vi "setTimebase.vi"(8 "error in (no error)":errorcluster, 9 "Delay [s]":dbl, 10 "Timebase [s/Div]":dbl, 11 "ScopeKeysight in":refnum<class "ScopeKeysight.lvclass">) -> (0 "error out":errorcluster, 3 "ScopeKeysight out":refnum<class "ScopeKeysight.lvclass">)   [LabVIEW 2023, in "ScopeKeysight.lvclass"]
doc: "<b>Author:</b> Wolfgang\n<b>Description:</b> Configure the timebase"
uses:
  ScopeKeysight.lvclass
  ScopeKeysight.lvclass/ScopeKeysight.ctl
  Driver/Public/Configure/Configure Timebase (Basic).vi
  Driver/Keysight-DSQx3014T.lvlib
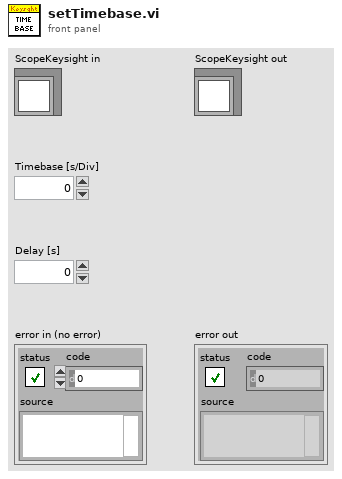
[diagram p1: front panel]
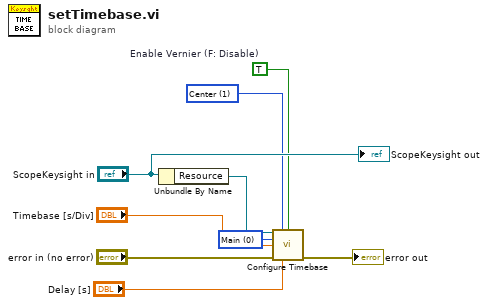
[diagram p0: block diagram]
diagram:
  w1 = 0 items=["Main", "Window", "XY", "Roll"] ("Time Base Type (0: Main)")
  w3 = TRUE  # Enable Vernier (F: Disable)
  w4 = 1 items=["Left", "Center", "Right"] ("Reference (1: Center)")
  n1 = Unbundle By Name("ScopeKeysight in") -> ("Resource"=w9:refnum<visa-resource-name>)
  n2 = call-poly "Configure Timebase.vi"("VISA resource name"=w9, "Reference (1: Center)"=w4, "Enable Vernier (F: Disable)"=w3, "Time Base Type (0: Main)"=w1, "Scale (50 s/div)"="Timebase [s/Div]", "error in (no error)"="error in (no error)", "Position (0.0)"="Delay [s]") -> ("error out"=→"error out":errorcluster)  [unwired: 7 in, 1 out]
  "ScopeKeysight out" <- "ScopeKeysight in"
